vi "Log Message.vi"(8 "error in":errorcluster, 10 "MSG In":string, 11 "session in":T1) -> (0 "error out":errorcluster, 3 "session out":T1)   [LabVIEW 2015, in "System Log.lvclass"]
uses:
  System Log.lvclass
  _Session Fwk/Typedefs/Session Handle.ctl
  _Session Fwk/Session - Root.lvclass
  Controls/DVR.ctl
  System Log.lvclass/System Log.ctl
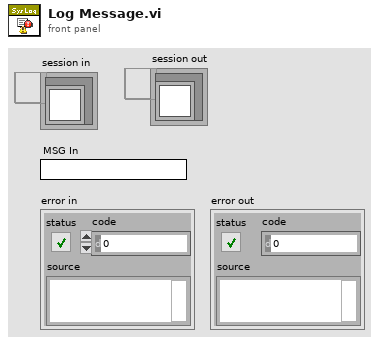
[diagram p1: front panel]
types:
  T1 = typedef "Session - Root.lvclass/Session Handle.ctl" = refnum<data-value>
  T2 = typedef "System Log.lvclass/DVR.ctl" = refnum<data-value>
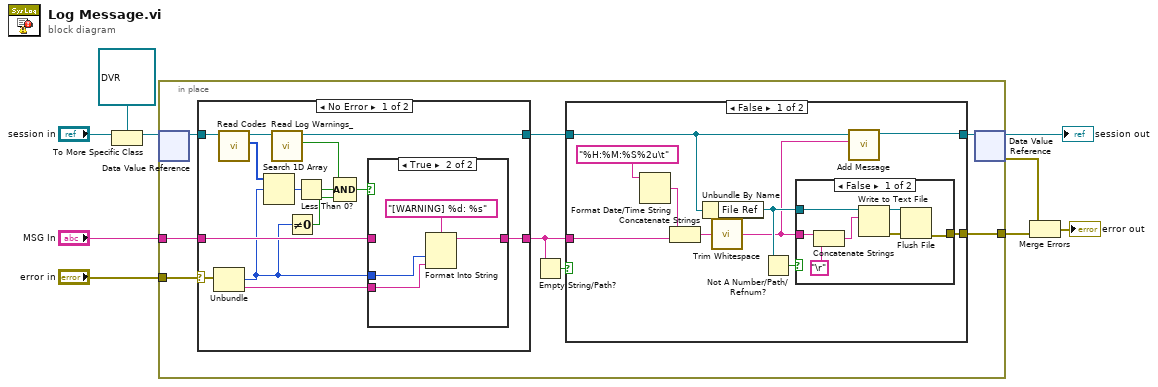
[diagram p0: block diagram]
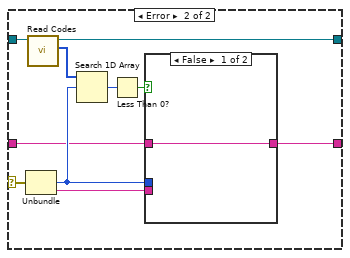
[diagram p5: hidden frame]
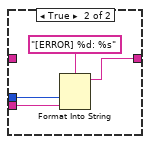
[diagram p6: hidden frame]
diagram:
  n1 = To More Specific Class(target class=T2 refnum ("DVR"), reference="session in") -> (specific class reference=w4:T2)  [unwired: 1 in, 1 out]
  n2 = in-place {
    in-place-border: "error in" -> [w17]
    in-place-border: "MSG In" -> [w16]
    in-place-border: [w12] -> w6
    n3 = in-place-dvr #1(w4) -> (w11:refnum<class "System Log.lvclass">)  [unwired: 1 out]
    n4 = case shown="No Error" w17 {
      selector: w17 -> [w46 w64]
      tunnel: w16 -> [w44 w55]
      tunnel: [w45 w62] -> w13
      tunnel: w11 -> [w49 w61]
      tunnel: [w42 w60] -> w10
      frame No Error {
        n5 = Unbundle(w46) -> ("code"=w38:i32, "source"=w36:string)  [unwired: 1 out]
        n6 = call "Read Codes.vi"("System Log in"=w49) -> ("Codes"=w47:i32[], "System Log out"=w43:refnum<class "System Log.lvclass">)  [unwired: 8 in, 1 out]
        n7 = Search 1D Array(1D array=w47, element=w38) -> (index of element=w48:i32)  [unwired: 1 in]
        n8 = call "Read Log Warnings_.vi"("System Log in"=w43) -> ("Log Warnings?"=w41:bool, "System Log out"=w42:refnum<class "System Log.lvclass">)  [unwired: 8 in, 1 out]
        n9 = Not Equal To 0?(x=w38) -> (x != 0?=w39:bool)
        n10 = Less Than 0?(x=w48) -> (x < 0?=w40:bool)
        n11 = Compound Arithmetic op=AND(w41, w40, w39) -> (w37:bool)
        n12 = case shown="True" w37 {
          tunnel: [w50 w53] -> w45
          tunnel: w44 -> [w50 _]
          tunnel: w38 -> [_ w52]
          tunnel: w36 -> [_ w51]
          frame False {
          }
          frame True {
            n13 = Format Into String(format string="[WARNING] %d: %s", w52, w51) -> (resulting string=w53:string)  [unwired: 2 in, 1 out]
          }
        }
      }
      frame Error {
        n14 = Unbundle(w64) -> ("code"=w58:i32, "source"=w63:string)  [unwired: 1 out]
        n15 = call "Read Codes.vi"("System Log in"=w61) -> ("Codes"=w59:i32[], "System Log out"=w60:refnum<class "System Log.lvclass">)  [unwired: 8 in, 1 out]
        n16 = Search 1D Array(1D array=w59, element=w58) -> (index of element=w57:i32)  [unwired: 1 in]
        n17 = Less Than 0?(x=w57) -> (x < 0?=w56:bool)
        n18 = case shown="False" w56 {
          tunnel: w63 -> [_ w69]
          tunnel: [w65 w68] -> w62
          tunnel: w58 -> [_ w66]
          tunnel: w55 -> [w65 _]
          frame False {
          }
          frame True {
            n19 = Format Into String(format string="[ERROR] %d: %s", w66, w69) -> (resulting string=w68:string)  [unwired: 2 in, 1 out]
          }
        }
      }
    }
    n20 = Empty String/Path?(string/path=w13) -> (empty?=w15:bool)
    n21 = case shown="False" w15 {
      tunnel: w10 -> [w20 w35]
      tunnel: [w19 w35] -> w14
      tunnel: w13 -> [w22 _]
      tunnel: [w25 _] -> w12
      frame False {
        n22 = Format Date/Time String(time format string (%c)="%H:%M:%S%2u\t") -> (date/time string=w23:string)  [unwired: 2 in]
        n23 = Concatenate Strings(w23, w22) -> (w21:string)
        n24 = Unbundle By Name(w20) -> ("File Ref"=w27:refnum<file>)
        n25 = call <vilib>:"Trim Whitespace.vi"("string"=w21) -> ("trimmed string"=w18:string)  [unwired: 1 in]
        n26 = Not A Number/Path/Refnum?(number/path/refnum=w27) -> (NaN/Path/Refnum?=w26:bool)
        n27 = case shown="False" w26 {
          tunnel: w27 -> [w34 _]
          tunnel: w18 -> [w33 _]
          tunnel: [w28 _] -> w25
          frame False {
            n28 = Concatenate Strings(w33, "\r") -> (w31:string)
            n29 = Write to Text File(file (use dialog)=w34, text=w31) -> (refnum out=w30:refnum<file>, error out=w29:errorcluster)  [unwired: 2 in, 1 out]
            n30 = Flush File(refnum=w30, error in=w29) -> (error out=w28:errorcluster)  [unwired: 1 out]
          }
          frame True {
          }
        }
        n31 = call "Add Message.vi"("New Msg"=w18, "Sys Log in"=w20) -> ("Sys Log out"=w19:refnum<class "System Log.lvclass">)  [unwired: 8 in, 1 out]
      }
      frame True {
      }
    }
    n32 = in-place-dvr #1(w14) -> (→"session out":T2, w7:errorcluster)
  }
  n33 = Merge Errors(w7, w6) -> (→"error out":errorcluster)
